vi "One Step Normalized.vi"(0 "m":u32[](array[numeric]), 1 "n-m":u32[](array[numeric]), 2 "table":dbl[][](array[numeric]) format="%.1f") -> (3 "m*":u32[](array[numeric]), 4 "n-m*":u32[](array[numeric]), 5 "table*":dbl[][](array[numeric]) format="%.1f", 6 "error":i32)   [LabVIEW 2010, in "NI_Gmath.lvlib"]
uses:
  NI_Gmath.lvlib
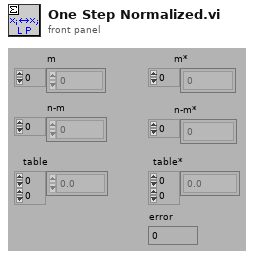
[diagram p1: front panel]
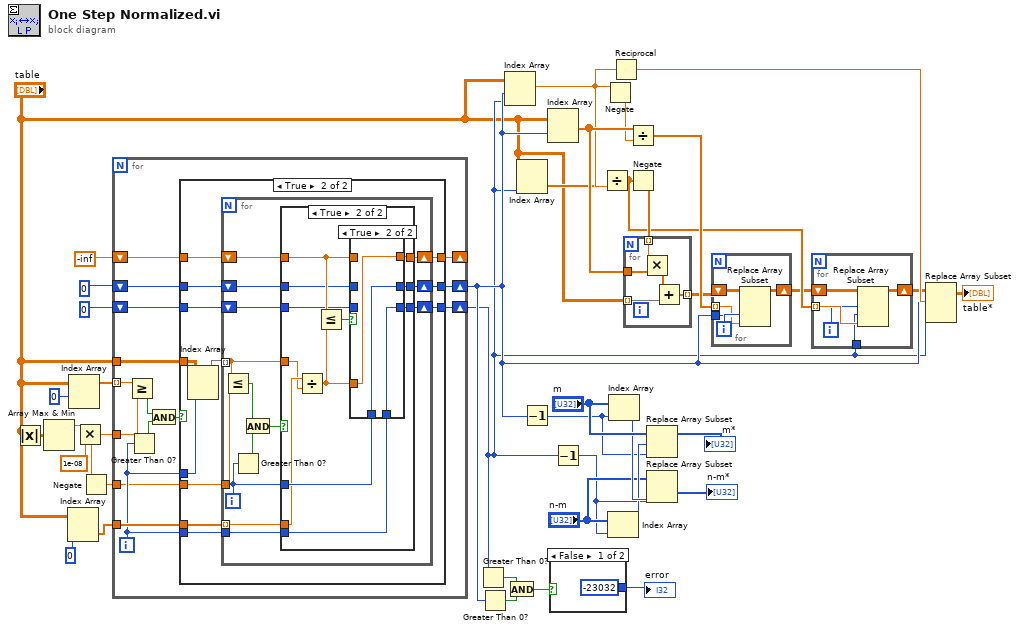
[diagram p0: block diagram]
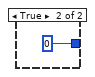
[diagram p2: hidden frame]
diagram:
  n1 = Absolute Value(x="table") -> (abs(x)=w4:dbl[][])
  n2 = Array Max & Min(array=w4) -> (max value=w6:dbl)  [unwired: 3 out]
  n3 = Index Array(array="table", index (col)=0) -> (element=w34:dbl[])  [unwired: 1 in]
  n4 = Index Array(array="table", index (row)=0) -> (element=w38:dbl[])  [unwired: 1 in]
  n5 = Multiply(x=w6, y=1e-08) -> (x*y=w2:dbl)
  n6 = Negate(x=w2) -> (-x=w1:dbl)
  n7 = for {
    tunnel: w38 -> [w42] mode=indexing
    tunnel: "table" -> [w44]
    shift-right: [w49] -> w12
    shift-left: 0 -> [w50]
    shift-right: [w47] -> w11
    shift-left: 0 -> [w48]
    tunnel: w34 -> [w51]
    shift-right: [w45] -> _
    shift-left: -inf -> [w46]
    tunnel: w2 -> [w41]
    tunnel: w1 -> [w40]
    i -> [w43]
    n8 = Greater Or Equal?(x=w42, y=w41) -> (x >= y?=w53:bool)
    n9 = Greater Than 0?(x=w43) -> (x > 0?=w54:bool)
    n10 = And(x=w53, y=w54) -> (x .and. y?=w52:bool)
    n11 = case shown="True" w52 {
      tunnel: w44 -> [_ w60]
      tunnel: w51 -> [_ w69]
      tunnel: w50 -> [w57 w68]
      tunnel: [w57 w66] -> w49
      tunnel: w48 -> [w56 w67]
      tunnel: [w56 w65] -> w47
      tunnel: w46 -> [w55 w64]
      tunnel: [w55 w63] -> w45
      tunnel: w43 -> [_ w62]
      tunnel: w43 -> [_ w59]
      tunnel: w40 -> [_ w58]
      frame False {
      }
      frame True {
        n12 = Index Array(array=w60, index (col)=w59) -> (element=w61:dbl[])  [unwired: 1 in]
        n13 = for {
          tunnel: w61 -> [w71] mode=indexing
          tunnel: w69 -> [w80] mode=indexing
          shift-right: [w78] -> w66
          shift-left: w68 -> [w79]
          shift-right: [w76] -> w65
          shift-left: w67 -> [w77]
          shift-right: [w74] -> w63
          shift-left: w64 -> [w75]
          tunnel: w62 -> [w72]
          tunnel: w58 -> [w70]
          i -> [w73]
          n14 = Less Or Equal?(x=w71, y=w70) -> (x <= y?=w82:bool)
          n15 = Greater Than 0?(x=w73) -> (x > 0?=w83:bool)
          n16 = And(x=w82, y=w83) -> (x .and. y?=w81:bool)
          n17 = case shown="True" w81 {
            tunnel: w71 -> [_ w88]
            tunnel: w80 -> [_ w89]
            tunnel: w79 -> [w86 w91]
            tunnel: [w86 w96] -> w78
            tunnel: w77 -> [w85 w90]
            tunnel: [w85 w94] -> w76
            tunnel: w75 -> [w84 w92]
            tunnel: [w84 w93] -> w74
            tunnel: w73 -> [_ w97]
            tunnel: w72 -> [_ w95]
            frame False {
            }
            frame True {
              n18 = Divide(x=w89, y=w88) -> (x/y=w87:dbl)
              n19 = Less Or Equal?(x=w92, y=w87) -> (x <= y?=w98:bool)
              n20 = case shown="True" w98 {
                tunnel: w97 -> [_ w104]
                tunnel: [w100 w104] -> w96
                tunnel: w95 -> [_ w103]
                tunnel: [w99 w103] -> w94
                tunnel: [w101 w102] -> w93
                tunnel: w87 -> [_ w102]
                tunnel: w92 -> [w101 _]
                tunnel: w91 -> [w100 _]
                tunnel: w90 -> [w99 _]
                frame False {
                }
                frame True {
                }
              }
            }
          }
        }
      }
    }
  }
  n21 = Greater Than 0?(x=w11) -> (x > 0?=w10:bool)
  n22 = Greater Than 0?(x=w12) -> (x > 0?=w9:bool)
  n23 = Index Array(array="table", index (row)=w12, index (col)=w11) -> (element=w27:dbl)
  n24 = And(x=w10, y=w9) -> (x .and. y?=w8:bool)
  n25 = Index Array(array="table", index (col)=w11) -> (element=w17:dbl[])  [unwired: 1 in]
  n26 = Decrement(x=w12) -> (x-1=w19:i32)
  n27 = Index Array(array="table", index (row)=w12) -> (element=w31:dbl[])  [unwired: 1 in]
  n28 = case shown="False" w8 {
    tunnel: [-23032 0] -> w7
    frame False {
    }
    frame True {
    }
  }
  "error" <- w7
  n29 = Decrement(x=w11) -> (x-1=w18:i32)
  n30 = Divide(x=w17, y=w27) -> (x/y=w28:dbl[])
  n31 = Negate(x=w27) -> (-x=w30:dbl)
  n32 = Index Array(array="n-m", index=w18) -> (element=w23:u32)
  n33 = Index Array(array="m", index=w19) -> (element=w24:u32)
  n34 = Reciprocal(x=w27) -> (1/x=w26:dbl)
  n35 = Divide(x=w31, y=w30) -> (x/y=w29:dbl[])
  n36 = Negate(x=w28) -> (-x=w32:dbl[])
  n37 = for {
    tunnel: "table" -> [w109] mode=indexing
    tunnel: w32 -> [w111] mode=indexing
    tunnel: w31 -> [w110]
    tunnel: [w107] -> w16 mode=indexing
    n38 = Multiply(x=w111, y=w110) -> (x*y=w108:dbl[])
    n39 = Add(x=w108, y=w109) -> (x+y=w107:dbl[])
  }
  n40 = Replace Array Subset(array="m", new element=w23, index=w19) -> (→"m*":u32[])
  n41 = Replace Array Subset(array="n-m", new element=w24, index=w18) -> (→"n-m*":u32[])
  n42 = for {
    tunnel: w12 -> [w115]
    tunnel: w29 -> [w114] mode=indexing
    shift-right: [w112] -> w15
    shift-left: w16 -> [w113]
    i -> [w116]
    n43 = Replace Array Subset(array=w113, new element=w114, index (row)=w115, index (col)=w116) -> (w112:dbl[][])
  }
  n44 = for {
    tunnel: w28 -> [w121] mode=indexing
    shift-right: [w119] -> w14
    shift-left: w15 -> [w120]
    tunnel: w11 -> [w117]
    i -> [w118]
    n45 = Replace Array Subset(array=w120, new element=w121, index (row)=w118, index (col)=w117) -> (w119:dbl[][])
  }
  n46 = Replace Array Subset(array=w14, new element=w26, index (row)=w12, index (col)=w11) -> (→"table*":dbl[][])
